vi "fgt set pressure.vi"(8 "error in (no error)":errorcluster, 10 "pressure":sgl, 11 "pressureIndex":u32) -> (0 "error out":errorcluster)   [LabVIEW 2016, in "fgt_SDK.lvlib"]
doc: "Send pressure command to selected device"
uses:
  fgt_SDK.lvlib
  dlls/fgt_SDK_32.dll
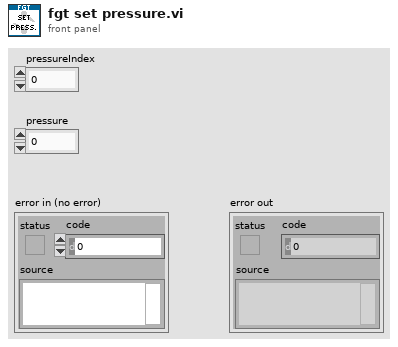
[diagram p1: front panel]
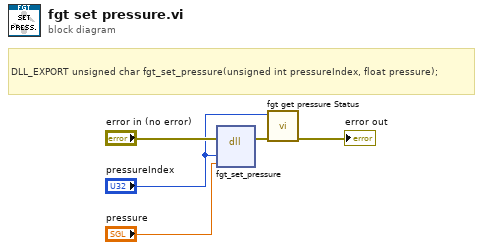
[diagram p0: block diagram]
diagram:
  # "DLL_EXPORT unsigned char fgt_set_pressure(unsigned int pressureIndex, float pressure);"
  n1 = dll-call lib="C:/projects/SDK/fgt-sdk-labview/dlls/fgt_SDK_*.*" fn="fgt_set_pressure"(error in="error in (no error)", "pressureIndex"="pressureIndex", "pressure"="pressure") -> (error out=w3:errorcluster)  [unwired: 5 in, 1 out]
  n2 = call "fgt get pressure Status.vi"("error in (no error)"=w3, "pressureIndex"="pressureIndex") -> ("error out"=→"error out":errorcluster)  [unwired: 9 in]
